vi "Ithaca pressure.vi"() -> (1 "Atmospheric pressure":dbl[unit], 2 "Atmospheric pressure (kPa)":dbl)   [LabVIEW 2012]
panel:
  in  "http URL":string="http://cuinfo.cornell.edu/Ithaca/Weather/"
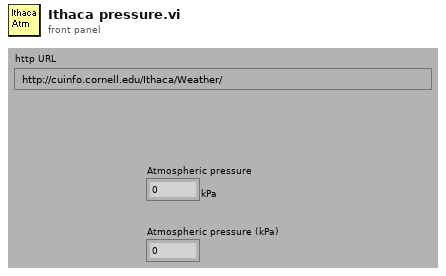
[diagram p1: front panel]
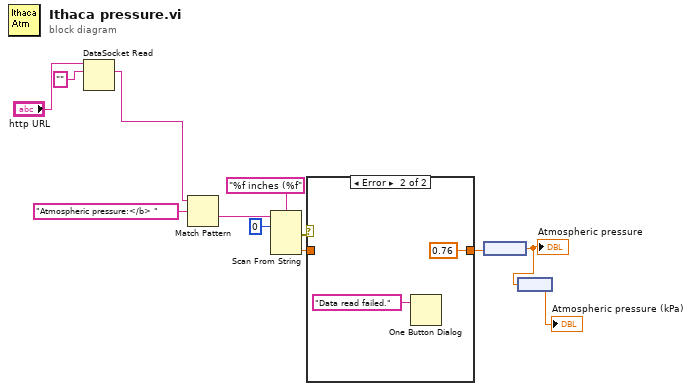
[diagram p0: block diagram]
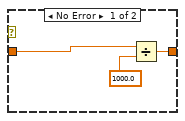
[diagram p2: hidden frame]
diagram:
  n1 = DataSocket Read(10:"" ("http URL"), 11:"http URL") -> (2:w2:string)  [unwired: 3 in, 6 out]
  n2 = Match Pattern(string=w2, regular expression="Atmospheric pressure:</b> ") -> (after substring=w9:string)  [unwired: 1 in, 3 out]
  n3 = Scan From String(format string="%f inches (%f", input string=w9, initial scan location=u32 0) -> (error out=w1:errorcluster, output 2=w8:dbl)  [unwired: 4 in, 2 out]
  n4 = case shown="Error" w1 {
    tunnel: w8 -> [w15 _]
    tunnel: [w13 0.76] -> w7
    frame No Error {
      n5 = Divide(x=w15, y=1000.0) -> (x/y=w13:dbl)
    }
    frame Error {
      n6 = One Button Dialog(message="Data read failed.") -> ()  [unwired: 1 in, 1 out]
    }
  }
  n7 = node(w7) -> (w5:dbl[unit])
  "Atmospheric pressure" <- w5
  n8 = node(w5) -> (→"Atmospheric pressure (kPa)":dbl)
